vi "root_Path.vi"() -> (3 "name or relative path":path=path "D:/PELUSO/ITSligo/lectures_MENG/5-Thesis/project")   [LabVIEW 2021, in "Framework_lib.lvlib"]
uses:
  QMH/Framework_lib.lvlib
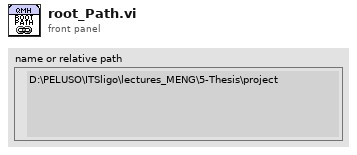
[diagram p1: front panel]
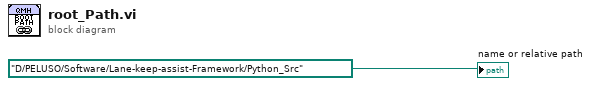
[diagram p0: block diagram]
diagram:
  "name or relative path" <- path "D:/PELUSO/Software/Lane-keep-assist-Framework/Python_Src" ("name or relative path")
